vi "MGI Bezier Inverse Multiple Solutions (DBL).vi"(1 "y":dbl format="%.2f", 2 "First k":i32, 3 "Bezier Control Points[]":dbl[](array[numeric]) format="%.4f") -> (0 "u[]":dbl[](array[numeric]) format="%.2f")   [LabVIEW 2020]
doc: "Calculates bezier 0..1 parameters from y, a bezier function result. All solutions in the range 0..1 are returned, in ascending order.\n\nAuthored by David A. Moore\nsupport@mooregoodideas.com\nwww.mooregoodideas.com\n\nCopyright (c) 2010, Moore Good Ideas, Inc.\n\nAll rights reserved.\n\nRedistribution and use in source and binary forms, with or without modification, are permitted provided that the following conditions are met:\n\n * Redistributions of source code must retain the above copyright notice, this list of conditions and the following disclaimer.\n * Redistributions in binary form must reproduce the above copyright notice, this list of conditions and the following disclaimer in the documentation and/or other materials provided with the distribution.\n * Neither the name of Moore Good Ideas, Inc. nor the names of its contributors may be used to endorse or promote products derived from this software without specific prior written permission.\n\nTHIS SOFTWARE IS PROVIDED BY THE COPYRIGHT HOLDERS AND CONTRIBUTORS \"AS IS\" AND ANY EXPRESS OR IMPLIED WARRANTIES, INCLUDING, BUT NOT LIMITED TO, THE IMPLIED WARRANTIES OF MERCHANTABILITY AND FITNESS FOR A PARTICULAR PURPOSE ARE DISCLAIMED. IN NO EVENT SHALL THE COPYRIGHT OWNER OR CONTRIBUTORS BE LIABLE FOR ANY DIRECT, INDIRECT, INCIDENTAL, SPECIAL, EXEMPLARY, OR CONSEQUENTIAL DAMAGES (INCLUDING, BUT NOT LIMITED TO, PROCUREMENT OF SUBSTITUTE GOODS OR SERVICES; LOSS OF USE, DATA, OR PROFITS; OR BUSINESS INTERRUPTION) HOWEVER CAUSED AND ON ANY THEORY OF LIABILITY, WHETHER IN CONTRACT, STRICT LIABILITY, OR TORT (INCLUDING NEGLIGENCE OR OTHERWISE) ARISING IN ANY WAY OUT OF THE USE OF THIS SOFTWARE, EVEN IF ADVISED OF THE POSSIBILITY OF SUCH DAMAGE."
panel:
  # "k"
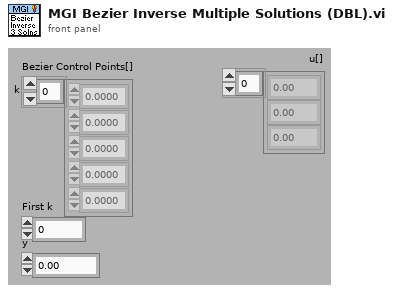
[diagram p1: front panel]
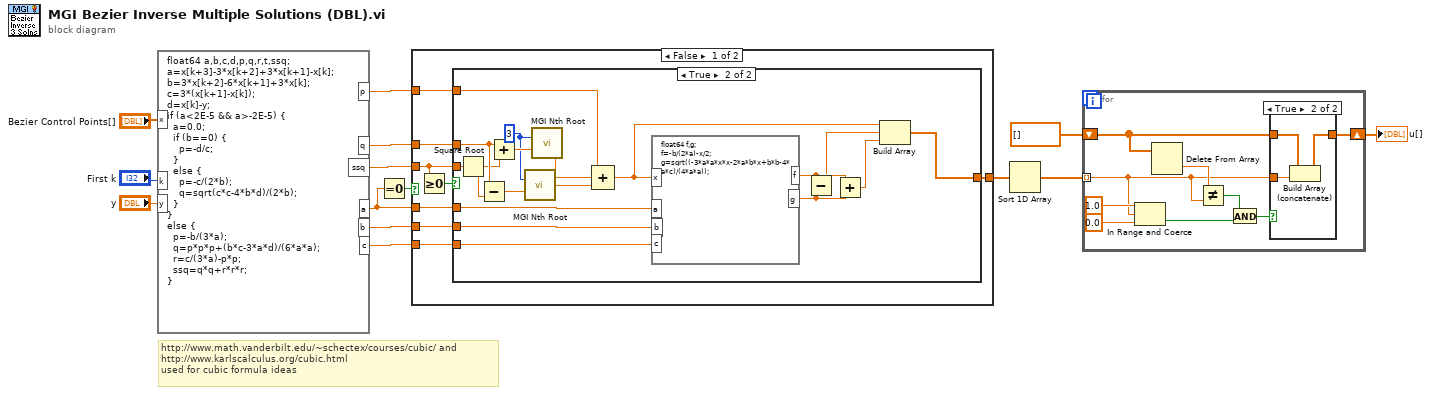
[diagram p0: block diagram]
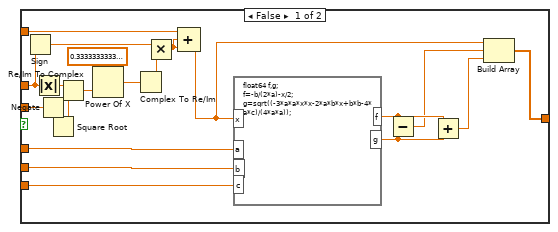
[diagram p2: hidden frame]
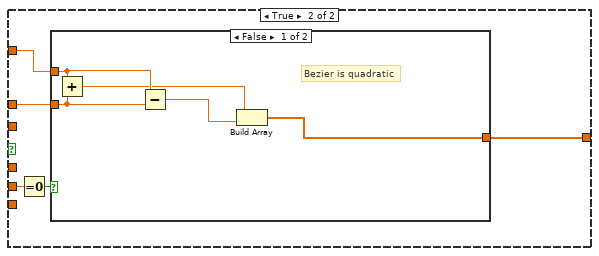
[diagram p3: hidden frame]
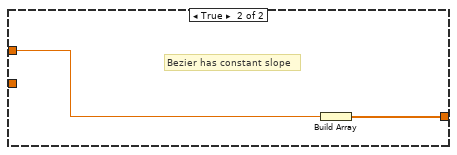
[diagram p4: hidden frame]
diagram:
  # "http://www.math.vanderbilt.edu/~schectex/courses/cubic/ and\nhttp://www.karlscalculus.org/cubic.html\nused for cubic formula ideas"
  n1 = formula code="float64 a,b,c,d,p,q,r,t,ssq;\na=x[k+3]-3*x[k+2]+3*x[k+1]-x[k];\nb=3*x[k+2]-6*x[k+1]+3*x[k];\nc=3*(x[k+1]-x[k]);\nd=x[k]-y;\nif (a<2E-5 && a>-2E-5) {\n  a=0.0;\n  if (b==0) {\n    p=-d/c;\n  }\n  else {\n    p=-c/(2*b);\n    q=sqrt(c*c-4*b*d)/(2*b);\n  }\n}\nelse {\n  p=-b/(3*a);\n  q=p*p*p+(b*c-3*a*d)/(6*a*a);\n  r=c/(3*a)-p*p;\n  ssq=q*q+r*r*r;\n}"("x"="Bezier Control Points[]", "y"="y", "k"="First k") -> ("p"=w7:dbl, "q"=w9:dbl, "ssq"=w8:dbl, "a"=w4:dbl, "b"=w5:dbl, "c"=w3:dbl)
  n2 = Equal To 0?(x=w4) -> (x = 0?=w6:bool)
  n3 = case shown="False" w6 {
    tunnel: w9 -> [w22 w66]
    tunnel: w8 -> [w19 _]
    tunnel: w7 -> [w21 w65]
    tunnel: [w20 w62] -> w11
    tunnel: w5 -> [w16 w64]
    tunnel: w4 -> [w17 _]
    tunnel: w3 -> [w15 _]
    frame False {
      n4 = Greater Or Equal To 0?(x=w19) -> (x >= 0?=w18:bool)
      n5 = case shown="True" w18 {
        tunnel: w22 -> [w36 w61]
        tunnel: w21 -> [w38 w54]
        tunnel: [w23 w44] -> w20
        tunnel: w19 -> [w43 w53]
        tunnel: w17 -> [w32 w52]
        tunnel: w16 -> [w31 w51]
        tunnel: w15 -> [w30 w50]
        frame False {
          n6 = Sign(1:w36) -> (0:w35:dbl)
          n7 = Absolute Value(x=w36) -> (abs(x)=w37:dbl)
          n8 = Negate(x=w43) -> (-x=w42:dbl)
          n9 = Square Root(x=w42) -> (sqrt(x)=w41:dbl)
          n10 = Re/Im To Complex(1:w41, 2:w37) -> (0:w40:cdb)
          n11 = Power Of X(1:w40, 2:cdb 0.3333333333333333-0.0i ("1/x")) -> (0:w39:cdb)
          n12 = Complex To Re/Im(x + iy=w39) -> (x=w34:dbl)  [unwired: 1 out]
          n13 = Multiply(x=w35, y=w34) -> (x*y=w33:dbl)
          n14 = Compound Arithmetic op=ADD(w38, w33, w33) -> (w26:dbl)
          n15 = formula code="float64 f,g;\nf=-b/(2*a)-x/2;\ng=sqrt((-3*a*a*x*x-2*a*b*x+b*b-4*a*c)/(4*a*a));"("x"=w26, "a"=w32, "b"=w31, "c"=w30) -> ("f"=w28:dbl, "g"=w27:dbl)
          n16 = Subtract(x=w28, y=w27) -> (x-y=w25:dbl)
          n17 = Add(x=w28, y=w27) -> (x+y=w24:dbl)
          n18 = Build Array(w26, w25, w24) -> (w23:dbl[])
        }
        frame True {
          w57 = 3 ("Root")
          n19 = Square Root(x=w53) -> (sqrt(x)=w60:dbl)
          n20 = Subtract(x=w61, y=w60) -> (x-y=w58:dbl)
          n21 = Add(x=w61, y=w60) -> (x+y=w59:dbl)
          n22 = call <userlib>:"MGI Nth Root.vi"("Root"=w57, "x"=w58) -> ("Numeric"=w56:dbl)  [unwired: 13 in]
          n23 = call <userlib>:"MGI Nth Root.vi"("Root"=w57, "x"=w59) -> ("Numeric"=w55:dbl)  [unwired: 13 in]
          n24 = Compound Arithmetic op=ADD(w54, w55, w56) -> (w47:dbl)
          n25 = formula code="float64 f,g;\nf=-b/(2*a)-x/2;\ng=sqrt((-3*a*a*x*x-2*a*b*x+b*b-4*a*c)/(4*a*a));"("x"=w47, "a"=w52, "b"=w51, "c"=w50) -> ("f"=w49:dbl, "g"=w48:dbl)
          n26 = Subtract(x=w49, y=w48) -> (x-y=w46:dbl)
          n27 = Add(x=w49, y=w48) -> (x+y=w45:dbl)
          n28 = Build Array(w47, w46, w45) -> (w44:dbl[])
        }
      }
    }
    frame True {
      n29 = Equal To 0?(x=w64) -> (x = 0?=w63:bool)
      n30 = case shown="False" w63 {
        tunnel: [w67 w72] -> w62
        tunnel: w66 -> [w71 _]
        tunnel: w65 -> [w70 w73]
        frame False {
          # "Bezier is quadratic"
          n31 = Add(x=w70, y=w71) -> (x+y=w69:dbl)
          n32 = Subtract(x=w70, y=w71) -> (x-y=w68:dbl)
          n33 = Build Array(w69, w68) -> (w67:dbl[])
        }
        frame True {
          # "Bezier has constant slope"
          n34 = Build Array(w73) -> (w72:dbl[])
        }
      }
    }
  }
  n35 = Sort 1D Array(array=w11) -> (sorted array=w2:dbl[])
  n36 = for {
    tunnel: w2 -> [w74] mode=indexing
    shift-right: [w79] -> w1
    shift-left: dbl[] [] ("u") -> [w78]
    n37 = In Range and Coerce(upper limit=1.0, x=w74, lower limit=0.0) -> (In Range?=w80:bool)  [unwired: 1 out]
    n38 = Delete From Array(array=w78) -> (deleted portion=w77:dbl)  [unwired: 2 in, 1 out]
    n39 = Not Equal?(x=w77, y=w74) -> (x != y?=w75:bool)
    n40 = And(x=w75, y=w80) -> (x .and. y?=w76:bool)
    n41 = case shown="True" w76 {
      tunnel: w74 -> [_ w84]
      tunnel: w78 -> [w83 w86]
      tunnel: [w83 w85] -> w79
      frame False {
      }
      frame True {
        n42 = Build Array (concatenate)(w86, w84) -> (w85:dbl[])
      }
    }
  }
  "u[]" <- w1
